vi "NXT_MIDBRAIN Left Wall Follow Behavior Data.vi"(1 "_sensorData":T2={"_irData"={"_irDistance"=0, "_irHeading"=0, "_irTimestamp"=0}, "_batteryVoltage"=0, "_NXTButtonStates"=[FALSE, FALSE, FALSE]}, 2 "Behavior #":i32, 3 "Previous Motor Position":T1={"_rudderCommand"=7, "_propCommand"=7, "_irServoCommand"=7}, 4 "Behavior Weights":T4=[0, 0, 0, 0, 0, 0]) -> (0 "Behavior Output":T5)   [LabVIEW 2012]
uses:
  behaviorOutput_t.ctl
  behaviorWeights_t.ctl
  sensorData_t.ctl
  irData_t.ctl
  motorCommands_t.ctl
panel:
  # "L\nE\nF\nT"
  # "C\nE\nN\nT\nE\nR"
  # "R\nI\nG\nH\nT"
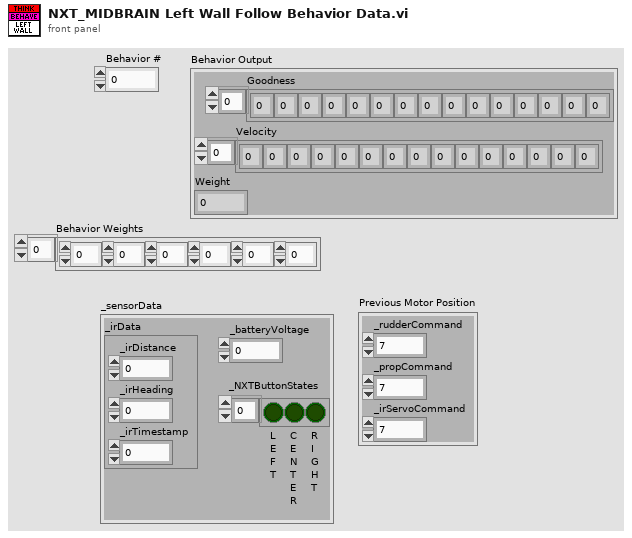
[diagram p1: front panel]
types:
  T1 = typedef "motorCommands_t.ctl" = cluster{"_rudderCommand":i8, "_propCommand":i8, "_irServoCommand":i8}
  T2 = typedef "sensorData_t.ctl" = cluster{"_irData":T3, "_batteryVoltage":i32, "_NXTButtonStates":bool[]}
  T3 = typedef "irData_t.ctl" = cluster{"_irDistance":i32, "_irHeading":i32, "_irTimestamp":u32}
  T4 = typedef "behaviorWeights_t.ctl" = i8[]
  T5 = typedef "behaviorOutput_t.ctl" = cluster{"Goodness":i8[], "Velocity":i8[], "Weight":i8}
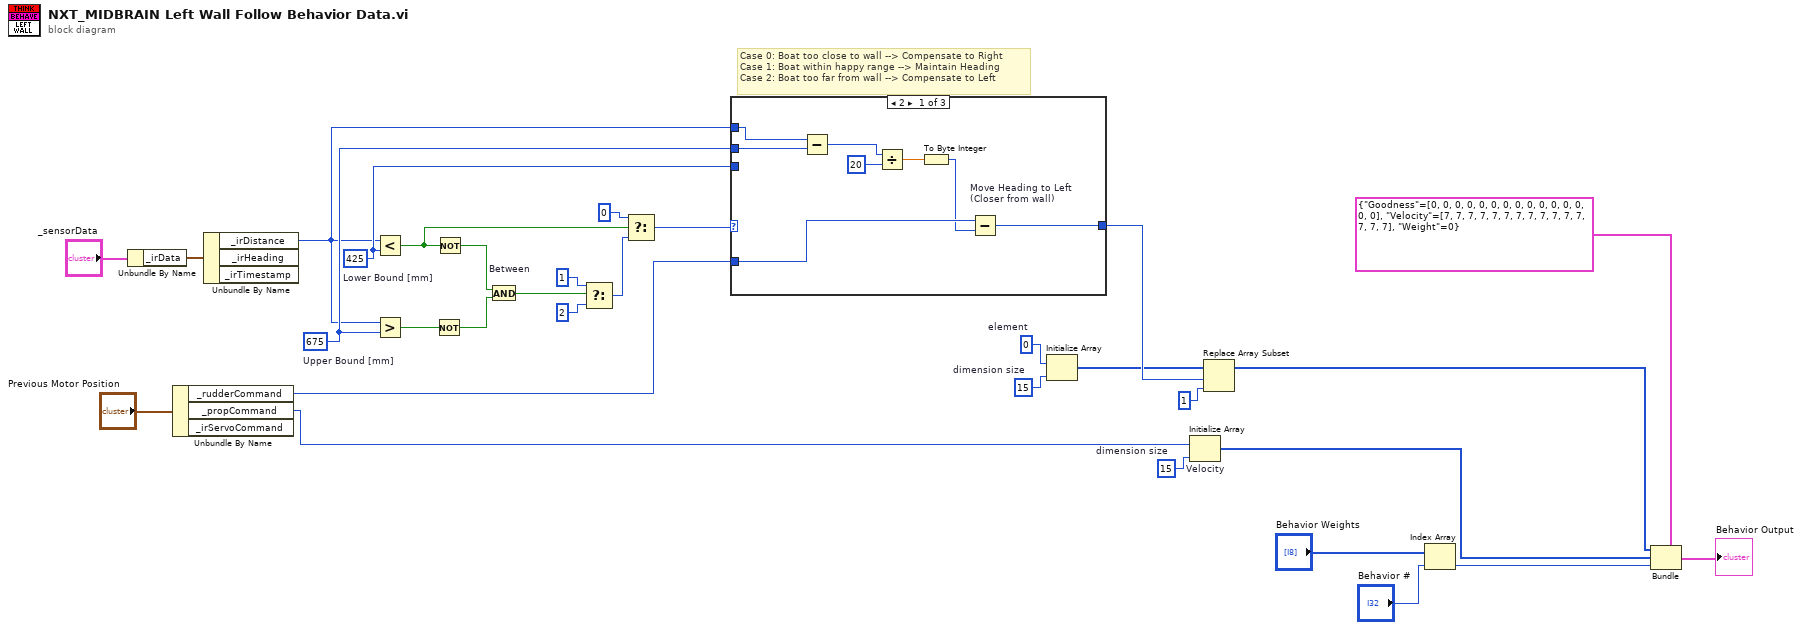
[diagram p0: block diagram]
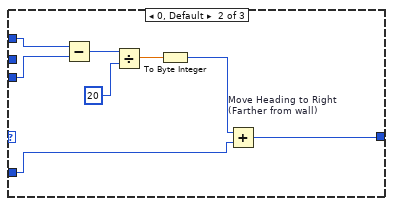
[diagram p2: hidden frame]
diagram:
  w3 = 15  # dimension size
  w6 = 15  # dimension size
  w7 = i8 0  # element
  w12 = 675  # Upper Bound [mm]
  w11 = 425  # Lower Bound [mm]
  # "Case 0: Boat too close to wall --> Compensate to Right\nCase 1: Boat within happy range --> Maintain Heading\nCase 2: Boat too far from wall --> Compensate to Left"
  n1 = Unbundle By Name("_sensorData") -> ("_irData"=w25:T3)
  n2 = Unbundle By Name("Previous Motor Position") -> ("_rudderCommand"=w13:i8, "_propCommand"=w2:i8)  [unwired: 1 out]
  n3 = Unbundle By Name(w25) -> ("_irDistance"=w10:i32)  [unwired: 2 out]
  n4 = Less?(x=w10, y=w11) -> (x < y?=w22:bool)
  n5 = Greater?(x=w10, y=w12) -> (0:w19:bool)
  n6 = Not(x=w19) -> (.not. x?=w23:bool)
  n7 = Not(x=w22) -> (.not. x?=w24:bool)
  n8 = And "Between"(x=w24, y=w23) -> (x .and. y?=w21:bool)
  n9 = Select(t=1, s=w21, f=2) -> (s? t:f=w20:i32)
  n10 = Select(t=0, s=w22, f=w20) -> (s? t:f=w15:i32)
  n11 = case shown="2" w15 {
    tunnel: w13 -> [w34 w45 w48]
    tunnel: [w32 w44 w48] -> w9
    tunnel: w12 -> [w38 _ _]
    tunnel: w11 -> [_ w46 _]
    tunnel: w10 -> [w39 w47 _]
    frame 2 {
      n12 = Subtract(x=w39, y=w38) -> (x-y=w37:i8)
      n13 = Divide(x=w37, y=i8 20) -> (x/y=w35:dbl)
      n14 = To Byte Integer(number=w35) -> (8bit integer=w33:i8)
      n15 = Subtract "Move Heading to Left\n(Closer from wall)"(x=w34, y=w33) -> (x-y=w32:i8)
    }
    frame 0, Default {
      n16 = Subtract(x=w47, y=w46) -> (x-y=w43:i32)
      n17 = Divide(x=w43, y=20) -> (x/y=w41:dbl)
      n18 = To Byte Integer(number=w41) -> (8bit integer=w40:i8)
      n19 = Add "Move Heading to Right\n(Farther from wall)"(x=w40, y=w45) -> (x+y=w44:i8)
    }
    frame 1 {
    }
  }
  n20 = Initialize Array(w7, w6) -> (w5:i8[])
  n21 = Initialize Array "Velocity"(w2, w3) -> (w1:i8[])
  n22 = Replace Array Subset(array=w5, new element=i8 1 ("new element/subarray"), index=w9) -> (w4:i8[])
  n23 = Index Array(array="Behavior Weights", index="Behavior #") -> (element=w27:i8)
  n24 = Bundle(cluster=T5 {"Goodness"=[0, 0, 0, 0, 0, 0, 0, 0, 0, 0, 0, 0, 0, 0, 0], "Velocity"=[7, 7, 7, 7, 7, 7, 7, 7, 7, 7, 7, 7, 7, 7, 7], "Weight"=0} ("Behavior Output"), "Goodness"=w4, "Velocity"=w1, "Weight"=w27) -> (→"Behavior Output":T5)
